vi "optionsAcq_gainAuto.vi"(0 "reference":refnum<class "OSA200.lvclass">, 2 "auto":bool, 4 "readWrite":enum16{"read", "write"}(ring), 5 "error in (no error)":errorcluster) -> (14 "duplicate reference":refnum<class "OSA200.lvclass">, 15 "status":string, 16 "auto out":bool, 19 "error out":errorcluster)   [LabVIEW 2010, in "OSA200.lvclass"]
uses:
  OSA200.lvclass
  OSA.lvclass
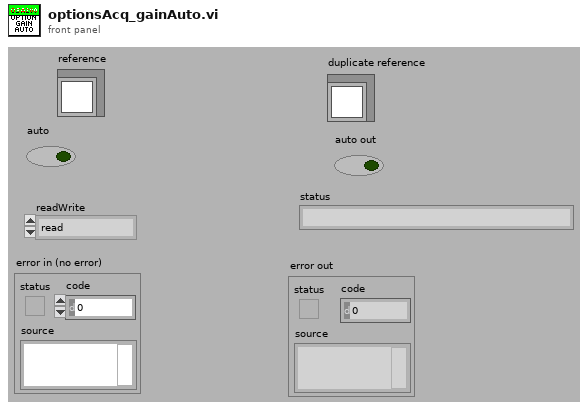
[diagram p1: front panel]
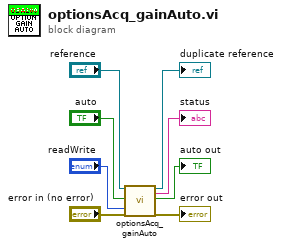
[diagram p0: block diagram]
diagram:
  n1 = call-parent "optionsAcq_gainAuto.vi"("reference"="reference", "auto"="auto", "readWrite"="readWrite", "error in (no error)"="error in (no error)") -> ("duplicate reference"=→"duplicate reference":refnum<class "OSA200.lvclass">, "status"=→"status":string, "auto out"=→"auto out":bool, "error out"=→"error out":errorcluster)  [unwired: 12 in]
